vi "GetKeyForPhraseLowLevel.vi"(7 "Dictionary":T1, 8 "error in (no error)":errorcluster, 11 "Phrase":string) -> (0 "error out":errorcluster, 3 "Key":string)   [LabVIEW 2020]
uses:
  Dictionary--Cluster.ctl
  Font -- Cluster.ctl
  Phrase Dictionary Entry -- Cluster.ctl
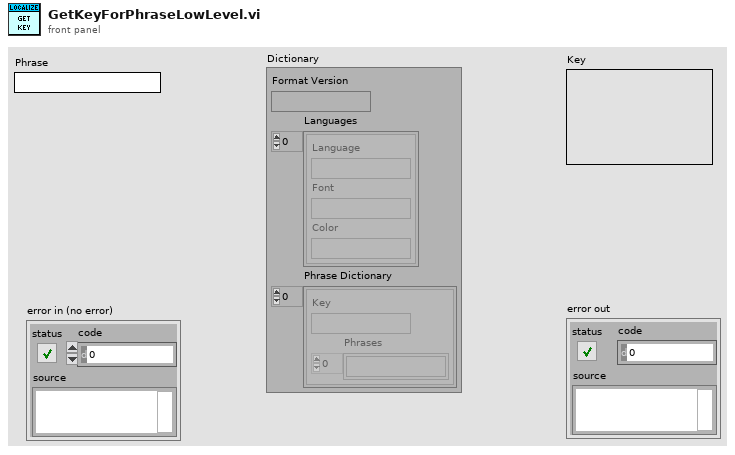
[diagram p1: front panel]
types:
  T1 = typedef "Dictionary--Cluster.ctl" = cluster{"Format Version":string, "Languages":T2[], "Phrase Dictionary":T3[]}
  T2 = typedef "Font -- Cluster.ctl" = cluster{"Language":string, "Font":string, "Color":string}
  T3 = typedef "Phrase Dictionary Entry -- Cluster.ctl" = cluster{"Key":string, "Phrases":string[]}
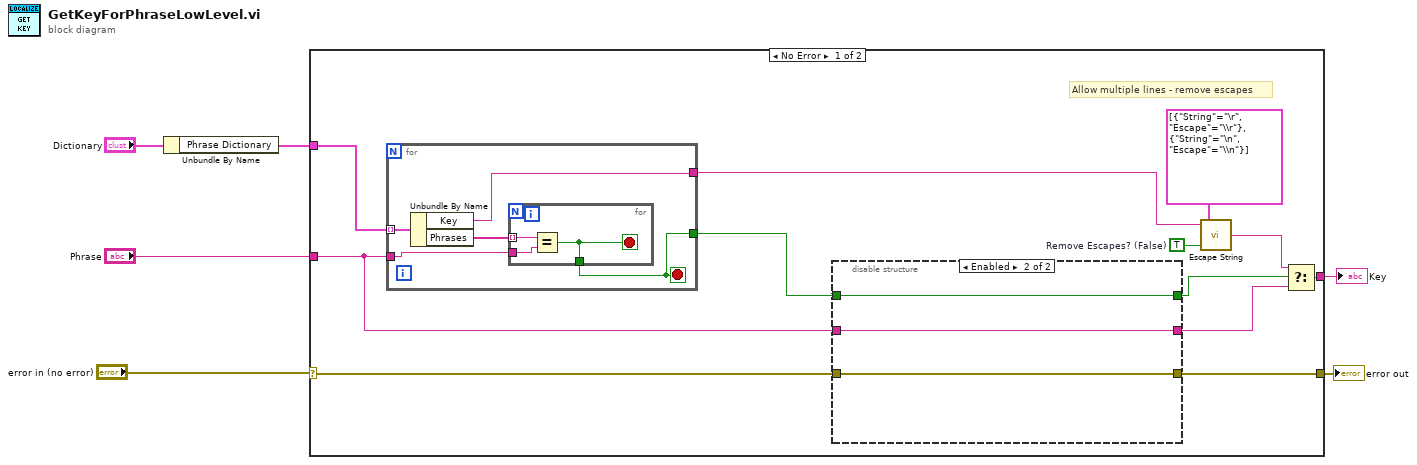
[diagram p0: block diagram]
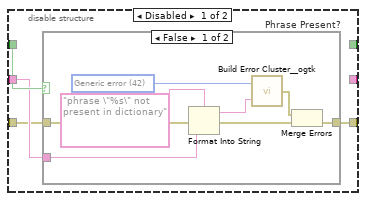
[diagram p2: hidden frame]
diagram:
  n1 = Unbundle By Name("Dictionary") -> ("Phrase Dictionary"=w1:T3[])
  n2 = case shown="No Error" "error in (no error)" {
    selector: "error in (no error)" -> [w11 w43]
    tunnel: [w13 _] -> w6
    tunnel: [w14 w43] -> w5
    tunnel: "Phrase" -> [w12 _]
    tunnel: w1 -> [w15 _]
    frame No Error {
      w18 = TRUE  # Remove Escapes? (False)
      # "Allow multiple lines - remove escapes"
      n3 = for {
        tunnel: w15 -> [w39] mode=indexing
        tunnel: w12 -> [w36]
        tunnel: [w38] -> w16
        tunnel: [w35] -> w10
        stop <- w38 stop-if-true
        n4 = Unbundle By Name(w39) -> ("Key"=w35:string, "Phrases"=w37:string[])
        n5 = for {
          tunnel: [w42] -> w38
          tunnel: w37 -> [w41] mode=indexing
          tunnel: w36 -> [w40]
          stop <- w42 stop-if-true
          n6 = Equal?(x=w41, y=w40) -> (x = y?=w42:bool)
        }
      }
      n7 = disable-structure shown="Enabled" {
        disable-tunnel: w16 -> [w22 w33]
        disable-tunnel: [w21 w34] -> w14
        disable-tunnel: w12 -> [w20 w32]
        disable-tunnel: w11 -> [w19 w34]
        disable-tunnel: [_ w33] -> w9
        disable-tunnel: [_ w32] -> w7
        frame Disabled {
          n8 = case "Phrase Present?" shown="False" w22 {
            tunnel: w19 -> [w27 w31]
            tunnel: [w28 w31] -> w21
            tunnel: w20 -> [w24 _]
            frame False {
              w30 = 42 items=["No error", "Argument error", "Memory is full", "Out of zone", "End of file", "File already open", "Generic file I/O error", "File not found", "File permission error", "Disk is full", "Duplicate path", "Too many files open", "System feature not enabled", "Resource file not found", "Cannot add resource", "Resource not found", "Image not found", "Image memory error", "Pen does not exist", "Config type invalid", "Config token not found", "Config parse error", "Config memory error", "Bad external code format", "Bad external code offset", "External code not present", "Null window", "Destroy window error", "Null menu", "Print aborted", "Bad print record", "Print driver error", "Windows error during printing", "Memory error during printing", "Print dialog error", "Generic print error", "Invalid device refnum", "Device not found", "Device parameter error", "Device unit error", "Cannot open device", "Device call aborted", "Generic error", "Cancelled by user", "Object ID too low", "Object ID too high", "Object not in heap", "Unknown heap", "Unknown object (invalid DefProc)", "Unknown object (DefProc not in table)", "Message out of range", "Invalid (null) method", "Unknown message", "Manager call not supported", "Bad address", "Network operation in progress", "Network operation timed out", "Connection is busy", "Network attribute not supported", "Network error", "Address in use", "System out of memory", "Connection aborted", "Connection refused", "Not connected", "Already connected", "Connection closed", "Initialization error (interapplication manager)", "Bad occurrence", "Wait on unbound occurrence handler", "Occurrence queue overflow", "Datalog type conflict", "Unused", "Unrecognized type (interapplication manager)", "Memory corrupt", "Failed to make temporary DLL", "Old CIN version", "Drag socket not found", "Failed to load drop-object", "Failed to register OLE object", "Failed to release OLE object", "Format specifier type mismatch", "Unknown format specifier", "Too few format specifiers", "Too many format specifiers", "Scan failed", "Newer CIN version", "Error converting to variant", "Runtime menu error", "Password tampered", "Variant attribute not found", "Incompatible variant data type", "Event data is not available", "Event Store is not present", "Occurrence is not found", "Event Queue is not created", "Event info is not available", "Refnum passed is NULL", "Error retrieving Class GUID", "Error retrieving CoClass GUID", "Error retrieving TypeLib GUID.", "Bad built application magic bytes.", "Specific driver is different from the specific driver associated with the Logical Name.", "There is no session opened to the class driver.", "Max Error", "MAX - Error with config objects", "MAX - Error loading configuration", "MAX - Group not supported"]
              n9 = Format Into String(format string="phrase \"%s\" not present in dictionary" ("String to Prepend to source (\"\")"), error in=w27, w24) -> (resulting string=w23:string, error out=w26:errorcluster)  [unwired: 1 in]
              n10 = call <userlib>:"Build Error Cluster__ogtk.vi"("String to Prepend to source (\"\")"=w23, "code"=w30) -> ("error out"=w29:errorcluster)
              n11 = Merge Errors(w29, w26) -> (w28:errorcluster)
            }
            frame True {
            }
          }
        }
        frame Enabled {
        }
      }
      n12 = call <vilib>:"Escape String.vi"("Remove Escapes? (False)"=w18, "Escapes"=cluster{"String":string, "Escape":string}[] [{"String"="\r", "Escape"="\\r"}, {"String"="\n", "Escape"="\\n"}], "String in"=w10) -> ("String out"=w8:string)
      n13 = Select(t=w8, s=w9, f=w7) -> (s? t:f=w13:string)
    }
    frame Error {
    }
  }
  "Key" <- w6
  "error out" <- w5
